vi "Pause.vi"(8 "error in (no error)":errorcluster, 11 "ASIA Pump C Settings in":T1) -> (0 "error out":errorcluster, 2 "Task Completed":bool=TRUE, 3 "ASIA Pump C Settings out":T1)   [LabVIEW 2018, in "ASIA Pump.lvlib"]
uses:
  ASIA Pump.lvlib
  Pump Settings.ctl
  Third Party Drivers/4600031 - Version 1.2-Asia Pump Drivers/AsiaPumpInterface.dll
  ASIA Support VIs.lvlib
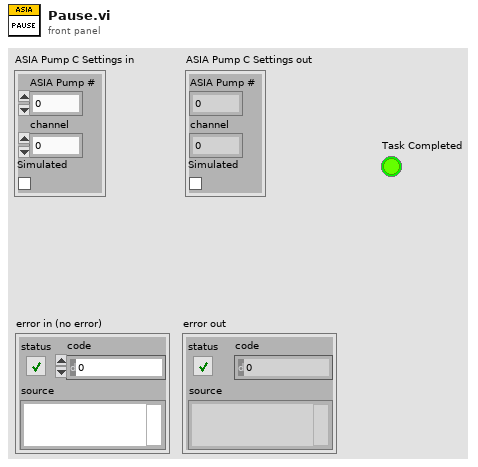
[diagram p1: front panel]
types:
  T1 = typedef "ASIA Pump.lvlib/Pump Settings.ctl" = cluster{"ASIA Pump #":i32, "channel":i32, "Simulated":bool}
  T2 = cluster{"Busy":bool, "PumpCnt":dbl, "RemoteEntered":bool, "OverpressureSet":bool}[]
  T3 = cluster{"Busy":bool, "PumpCnt":dbl, "RemoteEntered":bool, "OverpressureSet":bool}
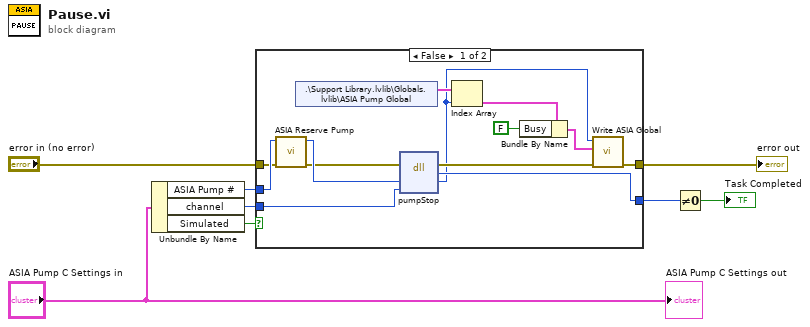
[diagram p0: block diagram]
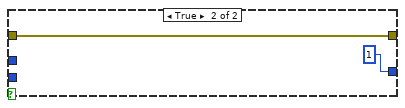
[diagram p2: hidden frame]
diagram:
  n1 = Unbundle By Name("ASIA Pump C Settings in") -> ("ASIA Pump #"=w7:i32, "channel"=w6:i32, "Simulated"=w2:bool)
  n2 = case shown="False" w2 {
    tunnel: w7 -> [w18 _]
    tunnel: w6 -> [w21 _]
    tunnel: "error in (no error)" -> [w14 w23]
    tunnel: [w17 w23] -> w4
    tunnel: [w20 u8 1 ("Bool")] -> w3
    frame False {
      n3 = call "ASIA Reserve Pump.vi"("error in (no error)"=w14, "ASIA Pump #"=w18) -> ("error out"=w15:errorcluster, "ASIA Pump #"=w19:i32)  [unwired: 8 in]
      n4 = shared-variable ".\\Support Library.lvlib\\Globals.lvlib\\ASIA Pump Global"() -> (w11:T2)  [unwired: 1 in, 1 out]
      n5 = dll-call lib="C:/Users/FAST Lab/Documents/LabVIEW Data/Projects/Pfizer Timed Seq/Third Party Drivers/4600031 - Version 1.2-Asia Pump Drivers/AsiaPumpInterface.dll" fn="pumpStop"(error in=w15, "pumpNum"=w19, "channel"=w21) -> (error out=w16:errorcluster, "Bool"=w20:u8, "pumpNum"=w9:u32)  [unwired: 3 in, 1 out]
      n6 = Index Array(array=w11, index=w9) -> (element=w10:T3)
      n7 = Bundle By Name(cluster=w10, "Busy"=FALSE) -> (w12:T3)
      n8 = call "Write ASIA Global.vi"("error in (no error)"=w16, "ASIA Global"=w12, "Pump Number"=w9) -> ("error out"=w17:errorcluster)  [unwired: 7 in, 1 out]
    }
    frame True {
    }
  }
  "error out" <- w4
  n9 = Not Equal To 0?(x=w3) -> (x != 0?=→"Task Completed":bool)
  "ASIA Pump C Settings out" <- "ASIA Pump C Settings in"
